vi "Read Config from File.vi"() -> ()   [LabVIEW 2014]
uses:
  Hardware/Table Stage/Controls/Translation Stage Cluster.ctl
  General/Controls/Translation Stage Types.ctl
  <vilib>/Utility/config.llb/NI_LVConfig.lvlib
panel:
  out "error out":errorcluster
  in  "error in (no error)":errorcluster
  in  "configuration file path":path
  in  "Control Param In":T1={"Position"=0.0, "Is.Enabled?"=FALSE, "Is.Connected?"=FALSE, "Device SN"="45876539", "AccelerationMaximum"=0.0, "VelocityMaximum"=0.0, "Acceleration"=0.0, "Velocity"=0.0, "waitTimeout (ms)"=0, "Model"=enum."None", "Is.Homed?"=FALSE}
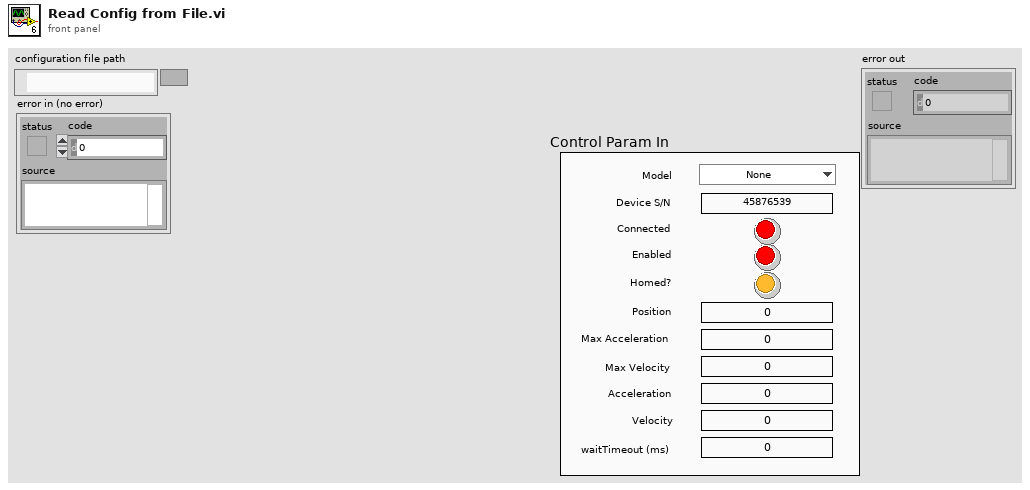
[diagram p1: front panel]
types:
  T1 = typedef "Translation Stage Cluster.ctl" = cluster{"Position":dbl, "Is.Enabled?":bool, "Is.Connected?":bool, "Device SN":string, "AccelerationMaximum":dbl, "VelocityMaximum":dbl, "Acceleration":dbl, "Velocity":dbl, "waitTimeout (ms)":i32, "Model":T2, "Is.Homed?":bool}
  T2 = typedef "Translation Stage Types.ctl" = enum16{"None", "Thorlabs LTS", "Thorlabs MLJ"}
  T3 = typedef "NI_LVConfig.lvlib/Config Data RefNum.ctl" = refnum<k1>
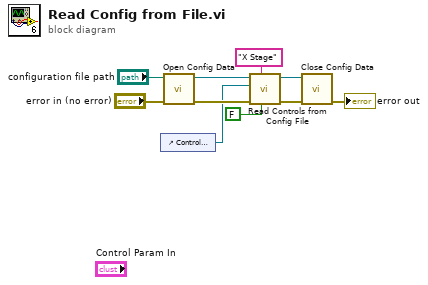
[diagram p0: block diagram]
diagram:
  n1 = control-ref of="Control Param In"() -> (w7:refnum<vi>)
  n2 = call <vilib>:"Open Config Data.vi"("error in (no error)"="error in (no error)", "configuration file path"="configuration file path") -> ("error out"=w10:errorcluster, "refnum"=w9:T3)  [unwired: 7 in, 1 out]
  n3 = call "Read Controls from Config File.vi"("Child?"=FALSE, "section"="X Stage", "Error In"=w10, "Ctl Refnum"=w7, "refnum"=w9) -> ("Error Out"=w5:errorcluster, "refnum out"=w4:T3)  [unwired: 5 in]
  n4 = call <vilib>:"Close Config Data.vi"("error in (no error)"=w5, "refnum"=w4) -> ("error out"=→"error out":errorcluster)  [unwired: 8 in, 1 out]
